vi "NXT-CAM-Dual.vi"() -> ()   [LabVIEW 2009]
uses:
  <vilib>/NXT/Subs/LVHSConnector.ctl
  <vilib>/NXT/Block Support/NXT_InputPort.ctl
  mindsensors.com LVEE Toolkit/Dual/NXTCam-DM.vi
panel:
  in  "Input of NXTCam":T1={"Tracking Mode"=0, "Object Number to Track"=0, "Address"=2} {"Address" format="%x"; "Object Number to Track" format="%x"; "Tracking Mode" items=["Disable Tracking", "Get First Object", "Get n th Object", "Enable Tracking", "Sort Objects  by size", "Sort Objects  by Colors", "Illumination on ", "Illumination Off", "Write Colormap", "Read Colormap", "Line tracking mode", "Object Tracking mode"]}
  out "Status \n(boolean)":bool
  in  "stop":bool
  out "NXT dup":T2={"error"={"status"=FALSE, "code"=0, "source"=""}, "address"="", "NXT #"=-1, "Show Error"=TRUE, "Connection"=4} caption="NXT" {"Connection" items=["USB", "Bluetooth", "USB then Bluetooth", "Last Connection", "Preference"]}
  out "Color":u8=1
  out "Y Upper Left":u8=80
  out "Y Lower Right":u8=113
  out "X Lower Right":u8=155
  in  "Input Port":T3 caption="Port (Port 4)" items=["Port 1", "Port 2", "Port 3", "Port 4"]
  in  "NXT":T2={"error"={"status"=FALSE, "code"=0, "source"=""}, "address"="", "NXT #"=-1, "Show Error"=TRUE, "Connection"=4} {"Connection" items=["USB", "Bluetooth", "USB then Bluetooth", "Last Connection", "Preference"]}
  out "X Upper Left":u8=108
  out "Total Objects":u8=8
  # "mindsensors.com\nCopyright (c) 2009 by mindsensors.com\nEmail: info (<at>) mindsensors (<dot>) com\n\nThis program is free software. You can redistribute it and/or modify\nit under the terms of the GNU General Public License as published by\nthe Free Software Foundation; version 3 of the License.\nRead the license at: http://www.gnu.org/licenses/gpl.txt"
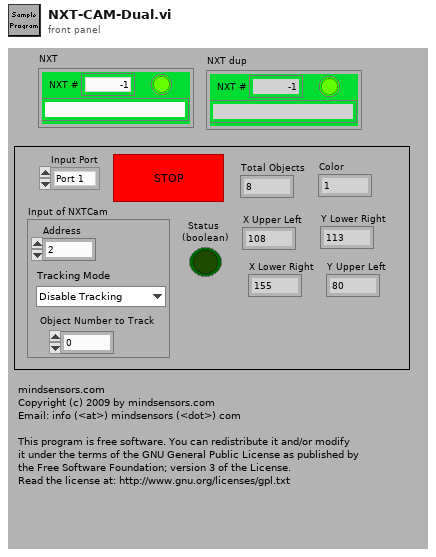
[diagram p1: front panel]
types:
  T1 = cluster{"Tracking Mode":u8, "Object Number to Track":u8, "Address":u8}
  T2 = typedef "LVHSConnector.ctl" = cluster{"error":errorcluster, "address":string, "NXT #":i32, "Show Error":bool, "Connection":u16}
  T3 = typedef "NXT_InputPort.ctl" = u8
  T4 = cluster{"Total Tracked Objects":u8, "Color":u8, "X Upper Left":u8, "Y Upper Left":u8, "X Lower Right":u8, "Y Lower Right":u8, "Status (boolean)":bool}
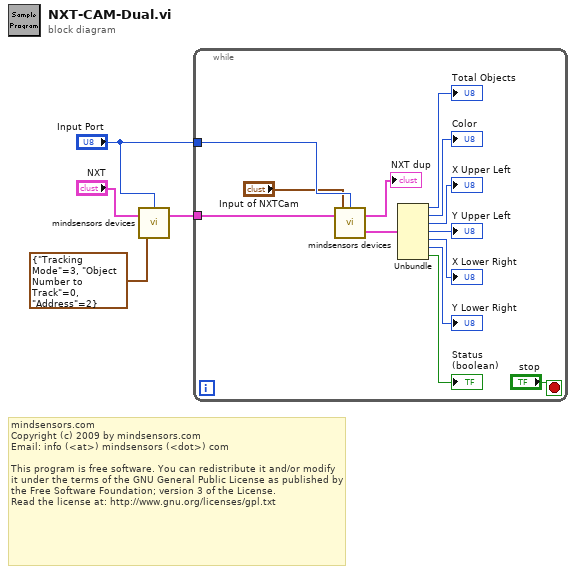
[diagram p0: block diagram]
diagram:
  # "mindsensors.com\nCopyright (c) 2009 by mindsensors.com\nEmail: info (<at>) mindsensors (<dot>) com\n\nThis program is free software. You can redistribute it and/or modify\nit under the terms of the GNU General Public License as published by\nthe Free Software Foundation; version 3 of the License.\nRead the license at: http://www.gnu.org/licenses/gpl.txt"
  n1 = call-poly "mindsensors devices.vi"("Input of NXTCam"=T1 {"Tracking Mode"=3, "Object Number to Track"=0, "Address"=2}, "NXT"="NXT", "Input Port"="Input Port") -> ("NXT dup"=w4:T2)  [unwired: 1 out]
  n2 = while {
    tunnel: w4 -> [w14]
    tunnel: "Input Port" -> [w13]
    stop <- "stop" stop-if-true
    n3 = call-poly "mindsensors devices.vi"("Input of NXTCam"="Input of NXTCam", "NXT"=w14, "Input Port"=w13) -> ("Output of NXTCam"=w17:T4, "NXT dup"=→"NXT dup":T2)
    n4 = Unbundle(w17) -> ("Total Tracked Objects"=→"Total Objects":u8, "Color"=→"Color":u8, "X Upper Left"=→"X Upper Left":u8, "Y Upper Left"=→"Y Upper Left":u8, "X Lower Right"=→"X Lower Right":u8, "Y Lower Right"=→"Y Lower Right":u8, "Status (boolean)"=→"Status \n(boolean)":bool)
  }
